vi "Compare ECAT FPGA.vi"(8 "error in (no error)":errorcluster, 10 "UDV Container in":refnum<k21>, 11 "FPGA in":T1 {"UDVs"."To FPGA"."VS ref" format="%.0x"; "UDVs"."From FPGA"."VS ref" format="%.0x"; "VS ref" format="%.0x"; "Output Data"."BD Refs"."Data Reference" format="%.0x"; "Input Data"."BD Refs"."Data Reference" format="%.0x"}) -> (0 "error out":errorcluster, 1 "Same?":bool, 2 "UDV Container out":refnum<k21>, 3 "FPGA out":T1 {"UDVs"."To FPGA"."VS ref" format="%.0x"; "UDVs"."From FPGA"."VS ref" format="%.0x"; "VS ref" format="%.0x"; "Output Data"."BD Refs"."Data Reference" format="%.0x"; "Input Data"."BD Refs"."Data Reference" format="%.0x"})   [LabVIEW 2015, in "Scan Engine Custom Device.lvlib"]
uses:
  Scan Engine Custom Device.lvlib
  Type Defs/FPGA Data.ctl
  <vilib>/NI Veristand/Custom Device API/Custom Device Item Ref.ctl
  Type Defs/Input Data.ctl
  <vilib>/NI Veristand/Custom Device API/Block Data Reference.ctl
  <vilib>/NI Veristand/Custom Device API/Data Reference.ctl
  Type Defs/Output Data.ctl
  Type Defs/UDV Data.ctl
  Type Defs/UDV Data Type.ctl
  Type Defs/FXP Config.ctl
  <resource>/objmgr/ni.var.rc
  <resource>/objmgr/IndComECAT.rc
  <vilib>/NI Veristand/Custom Device API/Custom Device API.lvlib
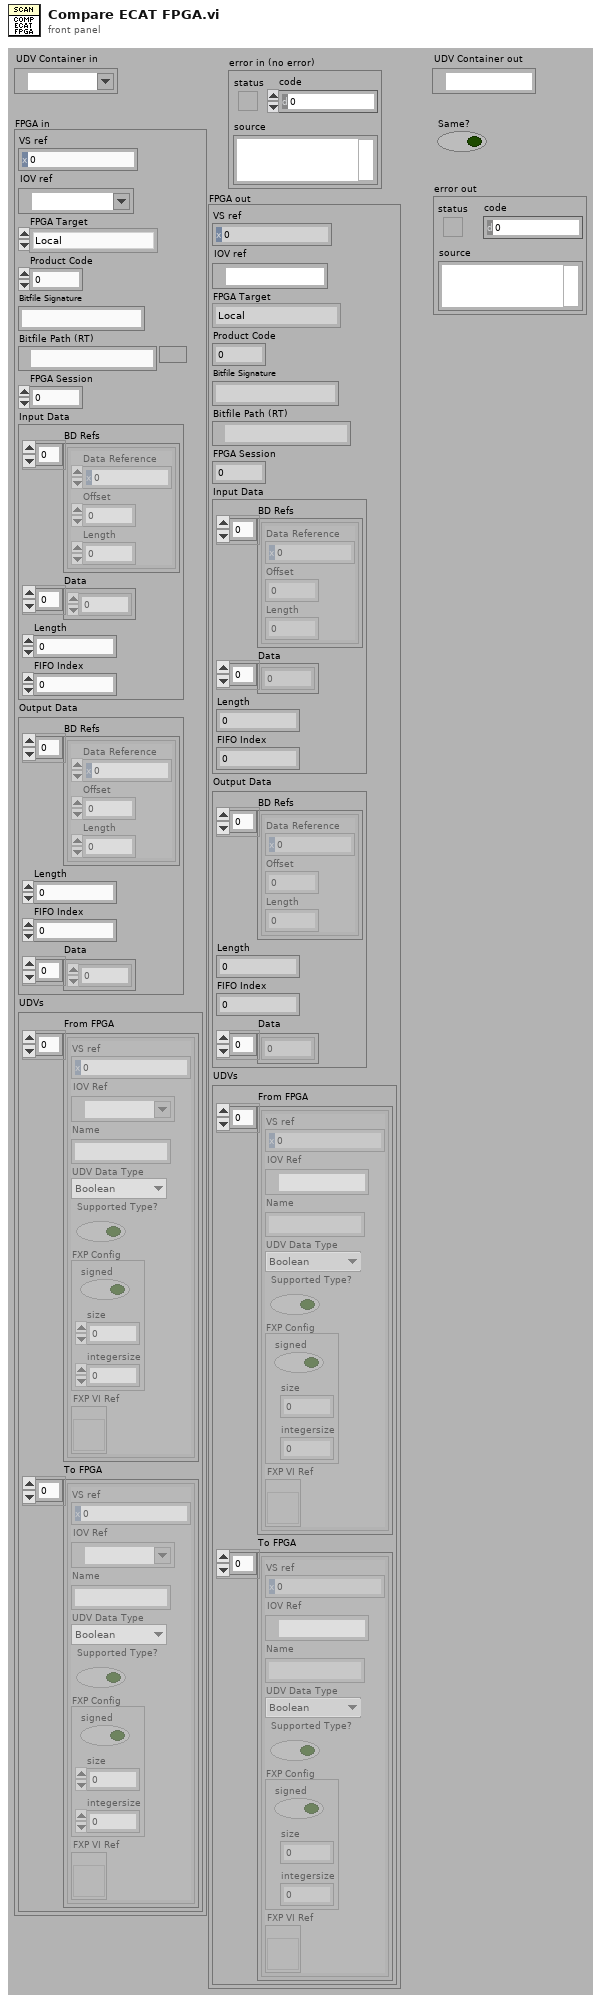
[diagram p1: front panel]
types:
  T1 = typedef "Scan Engine Custom Device.lvlib/FPGA Data.ctl" = cluster{"VS ref":T2, "IOV ref":refnum<k21>, "FPGA Target":enum16{"Local", "EtherCAT"}, "Product Code":u32, "Bitfile Signature":string, "Bitfile Path (RT)":path, "FPGA Session":u32, "Input Data":T3, "Output Data":T6, "UDVs":cluster{"From FPGA":T7[], "To FPGA":T7[]}}
  T2 = typedef "Custom Device API.lvlib/Custom Device Item Ref.ctl" = u64
  T3 = typedef "Scan Engine Custom Device.lvlib/Input Data.ctl" = cluster{"BD Refs":T4[], "Data":dbl[], "Length":i32, "FIFO Index":i32}
  T4 = typedef "Custom Device API.lvlib/Block Data Reference.ctl" = cluster{"Data Reference":T5, "Offset":u64, "Length":u64}
  T5 = typedef "Custom Device API.lvlib/Data Reference.ctl" = i32
  T6 = typedef "Scan Engine Custom Device.lvlib/Output Data.ctl" = cluster{"BD Refs":T4[], "Length":i32, "FIFO Index":i32, "Data":dbl[]}
  T7 = typedef "Scan Engine Custom Device.lvlib/UDV Data.ctl" = cluster{"VS ref":T2, "IOV Ref":refnum<k21>, "Name":string, "UDV Data Type":T8, "Supported Type?":bool, "FXP Config":T9, "FXP VI Ref":refnum<vi>}
  T8 = typedef "Scan Engine Custom Device.lvlib/UDV Data Type.ctl" = enum16{"Boolean", "Fixed Point", "Int8", "Int16", "Int32", "Int64", "U32 Bit Field", "UInt8", "UInt16", "UInt32", "UInt64", "Other"}
  T9 = typedef "Scan Engine Custom Device.lvlib/FXP Config.ctl" = cluster{"signed":bool, "size":u32, "integersize":i32}
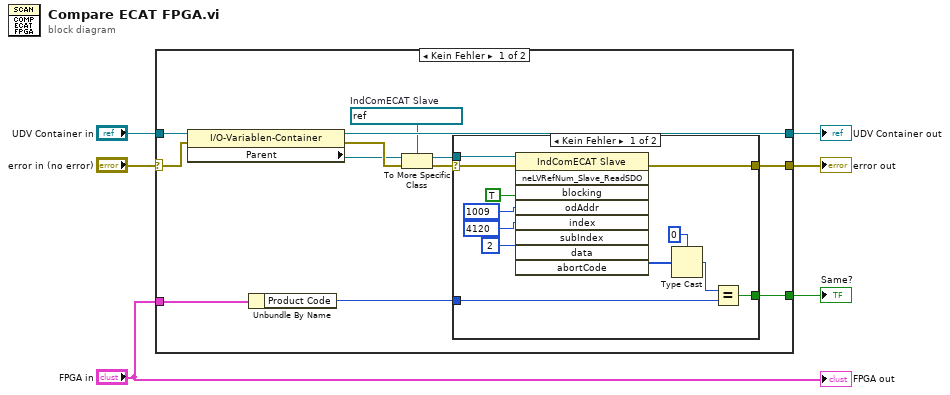
[diagram p0: block diagram]
diagram:
  n1 = case shown="Kein Fehler" "error in (no error)" {
    selector: "error in (no error)" -> [w7 w32]
    tunnel: [w18 w33] -> w6
    tunnel: [w17 w32] -> w5
    tunnel: "UDV Container in" -> [w11 w33]
    tunnel: [w10 _] -> w3
    tunnel: "FPGA in" -> [w8 _]
    frame No Error {
      w16 = refnum<k21> refnum  # IndComECAT Slave
      n2 = property class="I/O-Variablen-Container"(reference=w11, error in=w7) -> (reference out=w18:refnum<k21>, error out=w13:errorcluster, "Parent"=w12:refnum<k21>)
      n3 = Unbundle By Name(w8) -> ("Product Code"=w9:u32)
      n4 = To More Specific Class(target class=w16, reference=w12, error in=w13) -> (specific class reference=w15:refnum<k21>, error out=w14:errorcluster)
      n5 = case shown="Kein Fehler" w14 {
        selector: w14 -> [w20 w31]
        tunnel: w9 -> [w23 _]
        tunnel: [w22 _] -> w10
        tunnel: w15 -> [w21 _]
        tunnel: [w19 w31] -> w17
        frame No Error {
          n6 = invoke class="IndComECAT Slave" method="neLVRefNum_Slave_ReadSDO"(reference=w21, error in=w20, "blocking"=TRUE, "odAddr"=u16 1009, "index"=u16 4120, "subIndex"=u8 2) -> (error out=w19:errorcluster, "data"=w26:u8[])  [unwired: 3 in, 7 out]
          n7 = Type Cast(type=u32 0, x=w26) -> (*(type *) &x=w24:u32)
          n8 = Equal?(x=w24, y=w23) -> (x = y?=w22:bool)
        }
        frame Error {
        }
      }
    }
    frame Error {
    }
  }
  "UDV Container out" <- w6
  "error out" <- w5
  "Same?" <- w3
  "FPGA out" <- "FPGA in"
